vi "run.vi"(8 "error in (no error)":errorcluster, 9 "HWControllerEvents":refnum<class "HWControllerEvents.lvclass">, 10 "ChannelArray":refnum<class "ChannelArray.lvclass">, 11 "StaticOutputEditor":refnum<class "StaticOutputEditor.lvclass">) -> (0 "error out":errorcluster, 3 "StaticOutputEditor out":refnum<class "StaticOutputEditor.lvclass">)   [LabVIEW 2011, in "Views.lvlib" / "ScriptEditor.lvlib" / "StaticOutputEditor.lvclass"]
doc: "Runs the Static Hardware Controller viewer.\n\nUsed to manipulate hardware channels when script is not running.\nSends HWEvents to HWController."
uses:
  StaticOutputEditor.lvclass
  Hal/HWController/HWControllerEvents/HWControllerEvents.lvclass
  Tools/DatabaseHelpers/Database Objects/ChannelArray/ChannelArray.lvclass
  StaticOutputEditor.lvclass/StaticOutputEditor.ctl
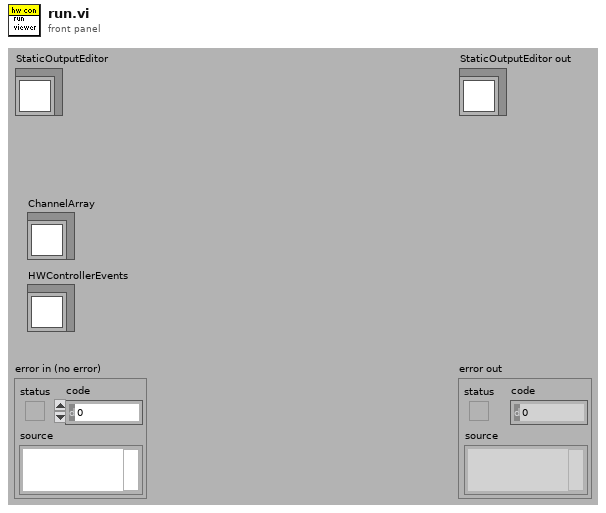
[diagram p1: front panel]
types:
  T1 = enum32{"Invalid", "Standard", "Closed", "Hidden", "Minimized", "Maximized"}
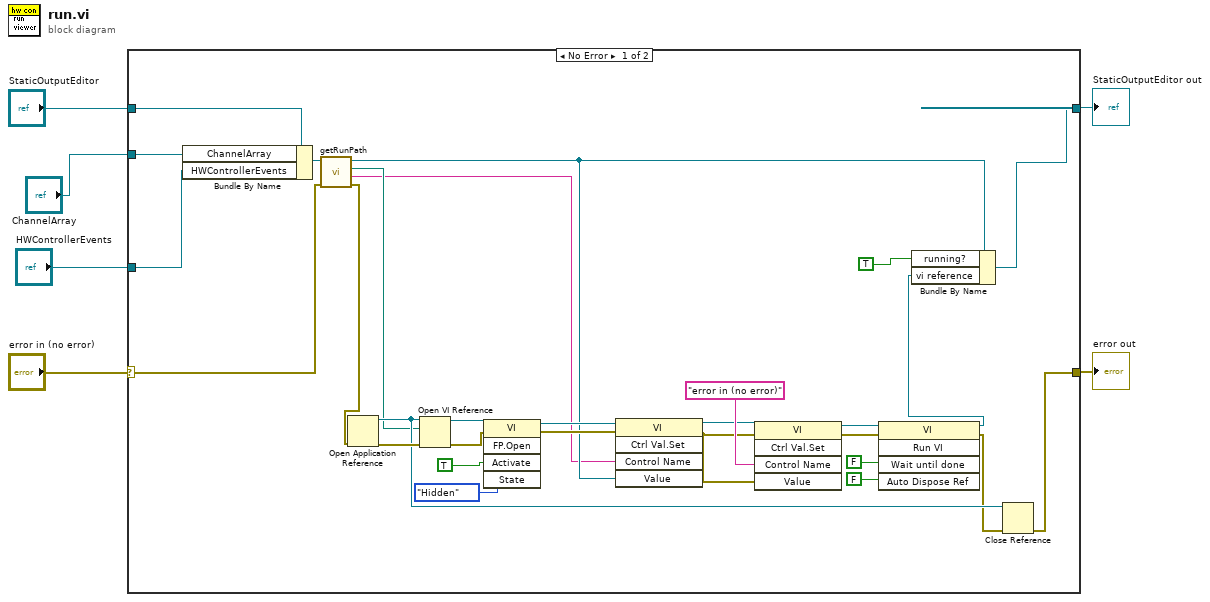
[diagram p0: block diagram]
diagram:
  n1 = case shown="No Error" "error in (no error)" {
    selector: "error in (no error)" -> [w7 w37]
    tunnel: [w23 w37] -> w5
    tunnel: [w27 w36] -> w3
    tunnel: "StaticOutputEditor" -> [w35 w36]
    tunnel: "HWControllerEvents" -> [w34 _]
    tunnel: "ChannelArray" -> [w13 _]
    frame No Error {
      n2 = Bundle By Name(cluster=w35, "ChannelArray"=w13, "HWControllerEvents"=w34) -> (w12:refnum<class "StaticOutputEditor.lvclass">)
      n3 = call-dynamic "getRunPath.vi"("error in (no error)"=w7, "StaticOutputEditor in"=w12) -> ("error out"=w10:errorcluster, "runParameter"=w8:string, "Path"=w9:path, "StaticOutputEditor out"=w11:refnum<class "StaticOutputEditor.lvclass">)  [unwired: 6 in]
      n4 = Open Application Reference(8:w10) -> (0:w30:errorcluster, 3:w25:refnum<vi>)  [unwired: 3 in]
      n5 = Open VI Reference(application reference (local)=w25, vi path=w9, error in (no error)=w30) -> (vi reference=w20:refnum<vi>, error out=w19:errorcluster)  [unwired: 3 in]
      n6 = invoke class="VI" method="FP.Open"(reference=w20, error in=w19, "Activate"=TRUE, "State"=T1."Hidden") -> (reference out=w18:refnum<vi>, error out=w17:errorcluster)  [unwired: 1 in, 3 out]
      n7 = invoke class="VI" method="Ctrl Val.Set"(reference=w18, error in=w17, "Control Name"=w8, "Value"=w11) -> (reference out=w29:refnum<vi>, error out=w28:errorcluster)  [unwired: 1 in, 3 out]
      n8 = invoke class="VI" method="Ctrl Val.Set"(reference=w29, error in=w28, "Control Name"="error in (no error)", "Value"=w28) -> (reference out=w22:refnum<vi>, error out=w21:errorcluster)  [unwired: 1 in, 3 out]
      n9 = invoke class="VI" method="Run VI"(reference=w22, error in=w21, "Wait until done"=FALSE, "Auto Dispose Ref"=FALSE) -> (reference out=w15:refnum<vi>, error out=w24:errorcluster)  [unwired: 1 in, 3 out]
      n10 = Bundle By Name(cluster=w11, "running?"=TRUE, "vi reference"=w15) -> (w27:refnum<class "StaticOutputEditor.lvclass">)
      n11 = Close Reference(reference=w25, error in (no error)=w24) -> (error out=w23:errorcluster)
    }
    frame Error {
    }
  }
  "error out" <- w5
  "StaticOutputEditor out" <- w3
